vi "Initialize Rx HW Channels for RT.vi"(5 "number of channels":i32=16, 9 "Rx Channels In":T2[](array[typedef])=[{"channel #"=0, "channel handle"=0, "labels settings for RT"=[]}, {"channel #"=0, "channel handle"=0, "labels settings for RT"=[]}, {"channel #"=0, "channel handle"=0, "labels settings for RT"=[]}, {"channel #"=0, "channel handle"=0, "labels settings for RT"=[]}] {"labels settings for RT"."Label Timestamp Channel Data Reference" format="%.0x"; "labels settings for RT"."Word Initial Raw Value" format="%032.0f"; "labels settings for RT"."Label Disable/Trigger Channel Reference" format="%.0x"; "labels settings for RT"."parameter driver data"."Tx parameter refs" format="%.0x"; "labels settings for RT"."SDI" format="%02b"; "labels settings for RT"."label" format="%.0o"}) -> (3 "Rx Channels Out":T2[](array[typedef]) {"labels settings for RT"."Label Timestamp Channel Data Reference" format="%.0x"; "labels settings for RT"."Word Initial Raw Value" format="%032.0f"; "labels settings for RT"."Label Disable/Trigger Channel Reference" format="%.0x"; "labels settings for RT"."parameter driver data"."Tx parameter refs" format="%.0x"; "labels settings for RT"."SDI" format="%02b"; "labels settings for RT"."label" format="%.0o"}, 4 "map from identifiers to indexes":T1)   [LabVIEW 2020, in "Ballard ARINC 429 Engine.lvlib" / "Custom Device.lvlib"]
uses:
  Custom Device.lvlib
  <vilib>/NI VeriStand/Custom Device API/Data Reference.ctl
  <vilib>/NI VeriStand/Custom Device API/Custom Device API.lvlib
  <vilib>/NI VeriStand/Custom Device API/Custom Device Item Ref.ctl
  Shared/Label.ctl
  Encoding and Decoding/Encoding.ctl
  Encoding and Decoding/Encoding and Decoding.lvlib
  Shared/Parameter Definition.ctl
  Shared/RT Parameters.ctl
  Shared/Transfer Type.ctl
  Shared/RT Label Settings.ctl
  Shared/RT Hardware Channel Settings.ctl
  Shared/Map of Identifiers to Indexes.ctl
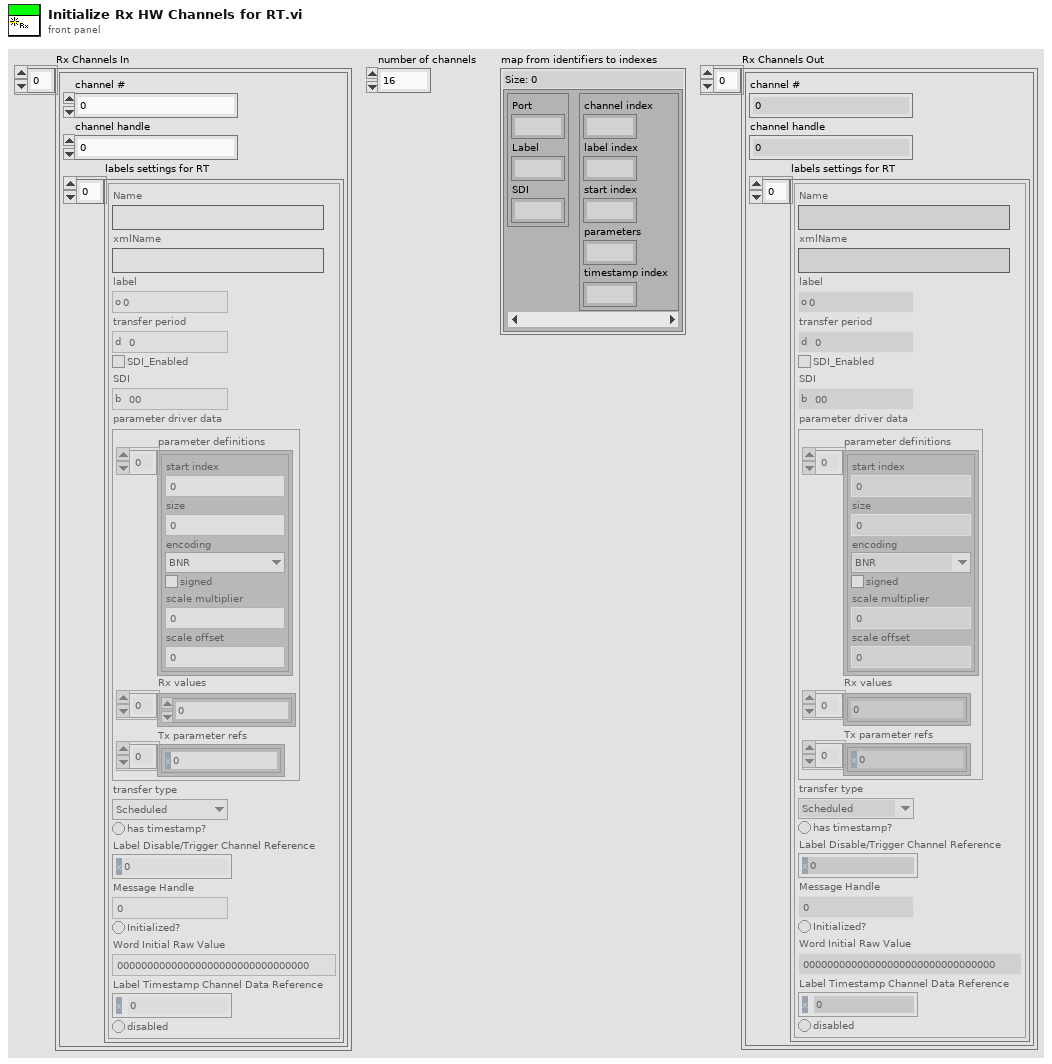
[diagram p1: front panel]
types:
  T1 = typedef "Map of Identifiers to Indexes.ctl" = map{cluster{"Port":u8, "Label":u8, "SDI":u8}, cluster{"channel index":i32, "label index":i32, "start index":i32, "parameters":i32, "timestamp index":i32}}
  T2 = typedef "RT Hardware Channel Settings.ctl" = cluster{"channel #":u16, "channel handle":u64, "labels settings for RT":T3[]}
  T3 = typedef "RT Label Settings.ctl" = cluster{"Name":string, "xmlName":string, "label":T4, "transfer period":u32, "SDI_Enabled":bool, "SDI":u8, "parameter driver data":T5, "transfer type":T9, "has timestamp?":bool, "Label Disable/Trigger Channel Reference":T8, "Message Handle":u64, "Initialized?":bool, "Word Initial Raw Value":u32, "Label Timestamp Channel Data Reference":T10, "disabled":bool}
  T4 = typedef "Label.ctl" = u8
  T5 = typedef "RT Parameters.ctl" = cluster{"parameter definitions":T6[], "Rx values":dbl[], "Tx parameter refs":T8[]}
  T6 = typedef "Parameter Definition.ctl" = cluster{"start index":i32, "size":i32, "encoding":T7, "signed":bool, "scale multiplier":dbl, "scale offset":dbl}
  T7 = typedef "Encoding and Decoding.lvlib/Encoding.ctl" = enum16{"BNR", "BCD", "Discrete"}
  T8 = typedef "Custom Device API.lvlib/Custom Device Item Ref.ctl" = u64
  T9 = typedef "Transfer Type.ctl" = enum16{"Scheduled", "Acyclic", "Block", "Strobe"}
  T10 = typedef "Custom Device API.lvlib/Data Reference.ctl" = i32
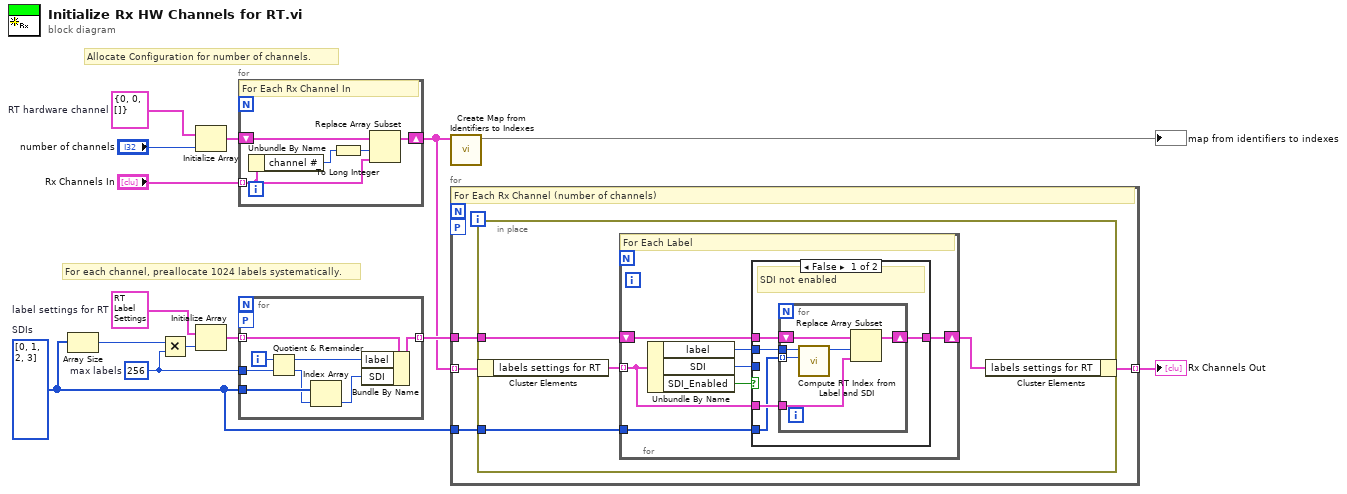
[diagram p0: block diagram]
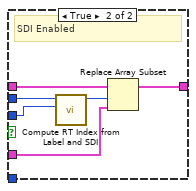
[diagram p2: hidden frame]
diagram:
  w8 = T2 {"channel #"=0, "channel handle"=0, "labels settings for RT"=[]}  # RT hardware channel
  w6 = 256  # max labels
  w13 = T3 {"Name"="", "xmlName"="", "label"=0, "transfer period"=0, "SDI_Enabled"=FALSE, "SDI"=0, "parameter driver data"={"parameter definitions"=[], "Rx values"=[], "Tx parameter refs"=[]}, "transfer type"=enum."Scheduled", "has timestamp?"=FALSE, "Label Disable/Trigger Channel Reference"=0, "Message Handle"=0, "Initialized?"=FALSE, "Word Initial Raw Value"=0, "Label Timestamp Channel Data Reference"=0, "disabled"=FALSE}  # label settings for RT
  w5 = u8[] [0, 1, 2, 3]  # SDIs
  # "For each channel, preallocate 1024 labels systematically."
  # "Allocate Configuration for number of channels."
  n1 = Array Size(array=w5) -> (size(s)=w10:i32)
  n2 = Multiply(x=w10, y=w6) -> (x*y=w12:i32)
  n3 = Initialize Array(w8, "number of channels") -> (w3:T2[])
  n4 = Initialize Array(w13, w12) -> (w11:T3[])
  n5 = for {
    tunnel: "Rx Channels In" -> [w16] mode=indexing
    shift-right: [w18] -> w2
    shift-left: w3 -> [w19]
    # "For Each Rx Channel In"
    n6 = Unbundle By Name(w16) -> ("channel #"=w17:u16)
    n7 = To Long Integer(number=w17) -> (32bit integer=w15:i32)
    n8 = Replace Array Subset(array=w19, new element=w16, index=w15) -> (w18:T2[])
  }
  n9 = for {
    tunnel: w11 -> [w25] mode=indexing
    tunnel: w6 -> [w26]
    tunnel: w5 -> [w24]
    tunnel: [w21] -> w9 mode=indexing
    workers-P: _ -> [_]
    i -> [w27]
    n10 = Quotient & Remainder(x=w27, y=w26) -> (x-y*floor(x/y)=w20:i32, floor(x/y)=w23:i32)
    n11 = Index Array(array=w24, index=w23) -> (element=w22:u8)
    n12 = Bundle By Name(cluster=w25, "label"=w20, "SDI"=w22) -> (w21:T3)
  }
  n13 = call "Create Map from Identifiers to Indexes.vi"("RT hardware channel data"=w2) -> ("map from identifiers to indexes"=→"map from identifiers to indexes":T1)  [unwired: 10 in]
  n14 = for {
    tunnel: w9 -> [w31]
    tunnel: w5 -> [w30]
    tunnel: w2 -> [w29] mode=indexing
    tunnel: [w28] -> w7 mode=indexing
    workers-P: _ -> [_]
    # "For Each Rx Channel (number of channels)"
    n15 = in-place {
      in-place-border: w31 -> [w35]
      in-place-border: w30 -> [w34]
      n16 = in-place-cluster #1(w29) -> ("labels settings for RT"=w33:T3[])
      n17 = for "Process each label" {
        tunnel: w33 -> [w40] mode=indexing
        shift-right: [w41] -> w32
        shift-left: w35 -> [w42]
        tunnel: w34 -> [w36]
        # "For Each Label"
        n18 = Unbundle By Name(w40) -> ("label"=w38:T4, "SDI"=w39:u8, "SDI_Enabled"=w37:bool)
        n19 = case shown="False" w37 {
          tunnel: w42 -> [w47 w59]
          tunnel: w40 -> [w44 w57]
          tunnel: w38 -> [w45 w56]
          tunnel: [w46 w58] -> w41
          tunnel: w39 -> [_ w55]
          tunnel: w36 -> [w43 _]
          frame False {
            # "SDI not enabled"
            n20 = for {
              tunnel: w45 -> [w49]
              tunnel: w44 -> [w51]
              shift-right: [w52] -> w46
              shift-left: w47 -> [w53]
              tunnel: w43 -> [w48] mode=indexing
              n21 = call "Compute RT Index from Label and SDI.vi"("SDI"=w48, "label"=w49) -> ("RT label index"=w50:i32)  [unwired: 9 in]
              n22 = Replace Array Subset(array=w53, new element=w51, index=w50) -> (w52:T3[])
            }
          }
          frame True {
            # "SDI Enabled"
            n23 = call "Compute RT Index from Label and SDI.vi"("SDI"=w55, "label"=w56) -> ("RT label index"=w54:i32)  [unwired: 9 in]
            n24 = Replace Array Subset(array=w59, new element=w57, index=w54) -> (w58:T3[])
          }
        }
      }
      n25 = in-place-cluster #1("labels settings for RT"=w32) -> (w28:T2)
    }
  }
  "Rx Channels Out" <- w7
